vi "Read P T_NTC.vi"(7 "cjc value":dbl=25.0 format="%0.2f") -> (0 "P Set 2 Output 2":dbl format="%.3g", 1 "P Set 1 Output 2":dbl format="%.3g", 2 "mean value P":dbl, 3 "String 2":string, 6 "termopar K":dbl format="%.3g", 8 "T Set 2 Output":dbl format="%.4g", 9 "T Set 1 Output":dbl format="%.4g", 10 "mean value T":dbl, 11 "String":string)   [LabVIEW 2011]
uses:
  <vilib>/Analysis/3filter.llb/Filter Passband Type.ctl
  <vilib>/DAQmx/read.llb/DAQmx Read (Analog 1D DBL 1Chan NSamp).vi
  <vilib>/DAQmx/create/channels.llb/DAQmx Create Channel (AI-Voltage-Basic).vi
  <vilib>/DAQmx/configure/timing.llb/DAQmx Timing (Sample Clock).vi
  <vilib>/DAQmx/miscellaneous.llb/DAQmx Fill In Error Info.vi
  <vilib>/Analysis/3filter.llb/Butterworth Filter (DBL).vi
  <vilib>/Analysis/baseanly.llb/Unimode.vi
  <vilib>/Analysis/5stat.llb/RMS (DBL).vi
  <vilib>/DAQmx/create/channels.llb/DAQmx Create Channel (AI-Temperature-Thermocouple).vi
  <vilib>/Analysis/NI_AALBase.lvlib
  Program Files/National Instruments/LabVIEW 2011/resource/objmgr/daqmx.rc
  <vilib>/gmath/NI_Gmath.lvlib
  <vilib>/Analysis/NI_AALPro.lvlib
panel:
  out "output variable":dbl
  in  "input C":dbl
  in  "input B":dbl
  in  "input A":dbl
  out "Rt":dbl
  in  "Vs":dbl
  in  "intervals 3":i32=20
  in  "Statistic 3":T1(ring)
  out "P Set 1 Output 3":dbl format="%.3g"
  out "?":T2(graph)
  out "Data Set 6":dbl[](graph)
  out "?":T2(graph)
  out "Data Set 5":dbl[](graph)
  out "error 3":dbl
  in  "filter type 3":T3
  in  "high cutoff freq: fh 3":dbl=0.45000000000000007 format="%0.2f"
  in  "low cutoff freq: fl 3":dbl=0.12500000000000006 format="%0.4f"
  in  "order 3":i32=2
  out "mean value P 2":dbl
  out "String 3":string
  in  "intervals 2":i32=20
  in  "Statistic 2":T1(ring)
  out "?":T2(graph)
  out "Data Set 4":dbl[](graph)
  out "?":T2(graph)
  out "Data Set 3":dbl[](graph)
  out "error 2":dbl
  in  "filter type 2":T3
  in  "high cutoff freq: fh 2":dbl=0.45000000000000007 format="%0.2f"
  in  "low cutoff freq: fl 2":dbl=0.12500000000000006 format="%0.4f"
  in  "order 2":i32=2
  in  "intervals":i32=20
  in  "Statistic":T1(ring)
  out "?":T2(graph)
  out "Data Set 1":dbl[](graph)
  out "?":T2(graph)
  out "Data Set 2":dbl[](graph)
  out "error":dbl
  in  "filter type":T3
  in  "high cutoff freq: fh":dbl=0.45000000000000007 format="%0.2f"
  in  "low cutoff freq: fl":dbl=0.12500000000000006 format="%0.4f"
  in  "order":i32=2
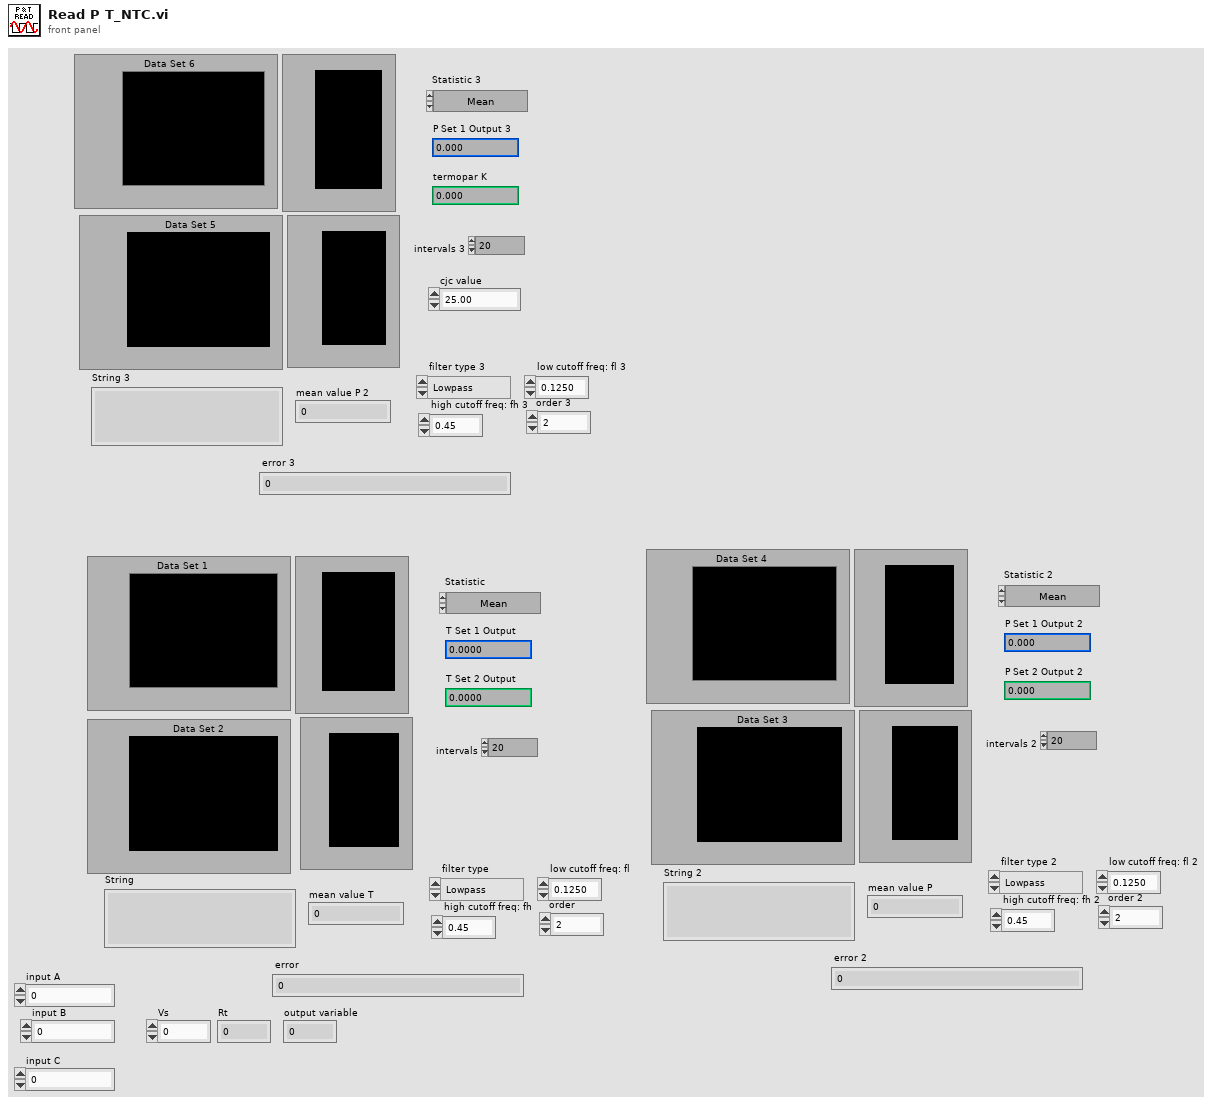
[diagram p1: front panel]
types:
  T1 = enum16{"Mean", "Standard Deviation", "Variance", "Skewness", "Kurtosis", "Median", "Mode", "RMS"}
  T2 = cluster{"Histogram: h(x)":i32[], "X Values":dbl[]}
  T3 = typedef "NI_AALBase.lvlib/Filter Passband Type.ctl" = enum32{"Lowpass", "Highpass", "Bandpass", "Bandstop"}
  T4 = enum16{"arithmetic", "geometric", "harmonic", "trimmed", "median"}
  T5 = cluster{"intervals":i32, "Statistic":enum16{"Mean", "Standard Deviation", "Variance", "Skewness", "Kurtosis", "Median", "Mode", "RMS"}}
  T6 = cluster{"intervals 2":i32, "Statistic 2":enum16{"Mean", "Standard Deviation", "Variance", "Skewness", "Kurtosis", "Median", "Mode", "RMS"}}
  T7 = cluster{"intervals 3":i32, "Statistic 3":enum16{"Mean", "Standard Deviation", "Variance", "Skewness", "Kurtosis", "Median", "Mode", "RMS"}}
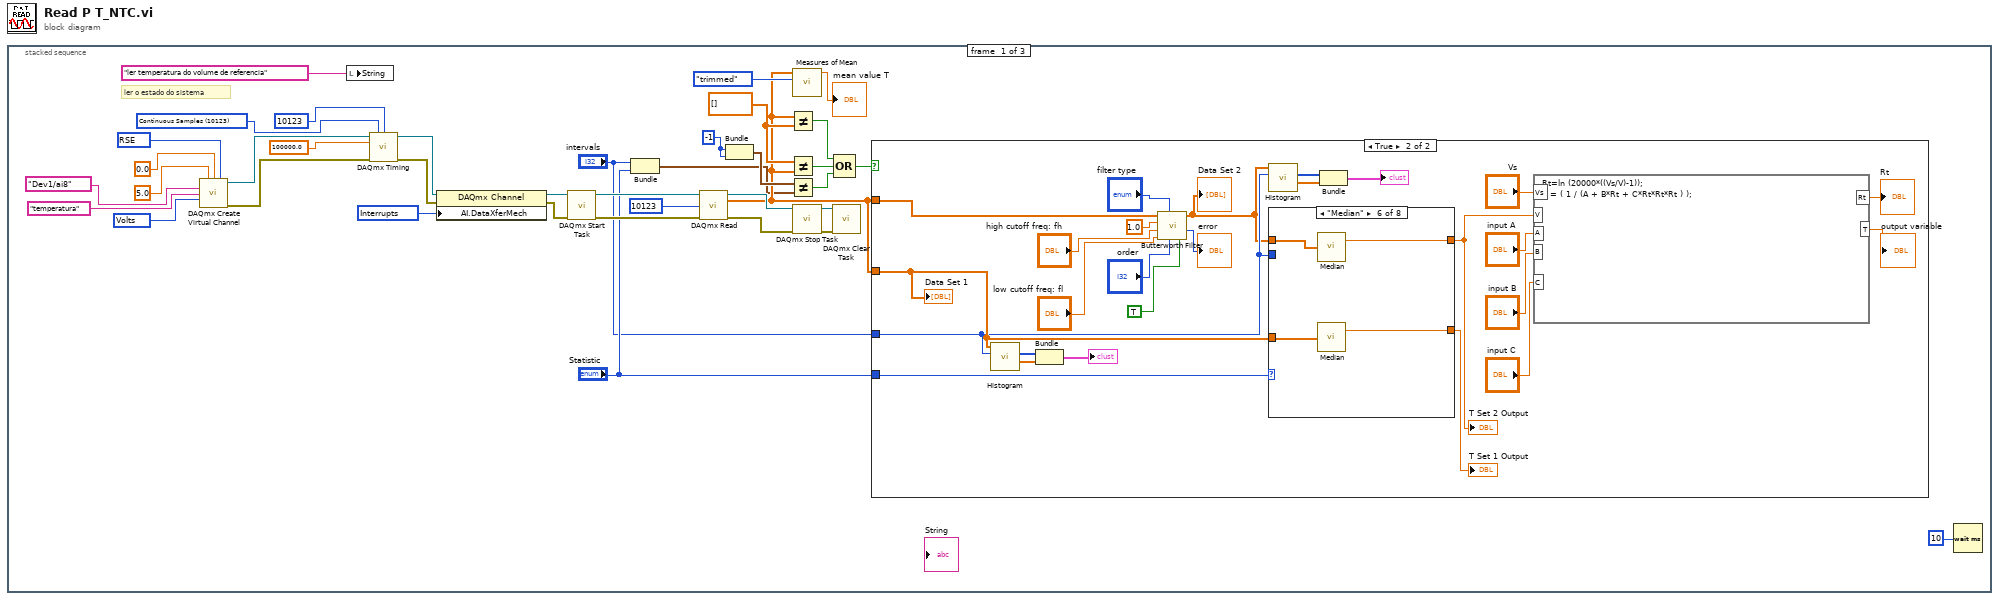
[diagram p0: block diagram]
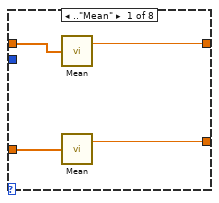
[diagram p3: hidden frame]
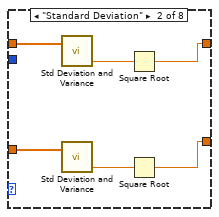
[diagram p4: hidden frame]
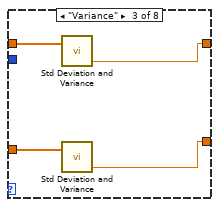
[diagram p5: hidden frame]
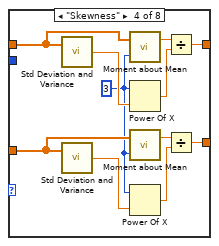
[diagram p6: hidden frame]
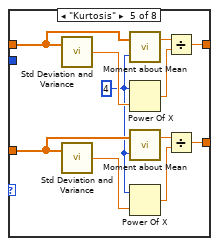
[diagram p7: hidden frame]
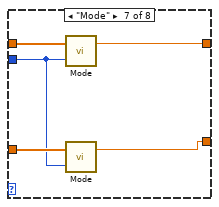
[diagram p8: hidden frame]
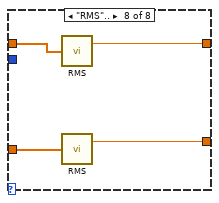
[diagram p9: hidden frame]
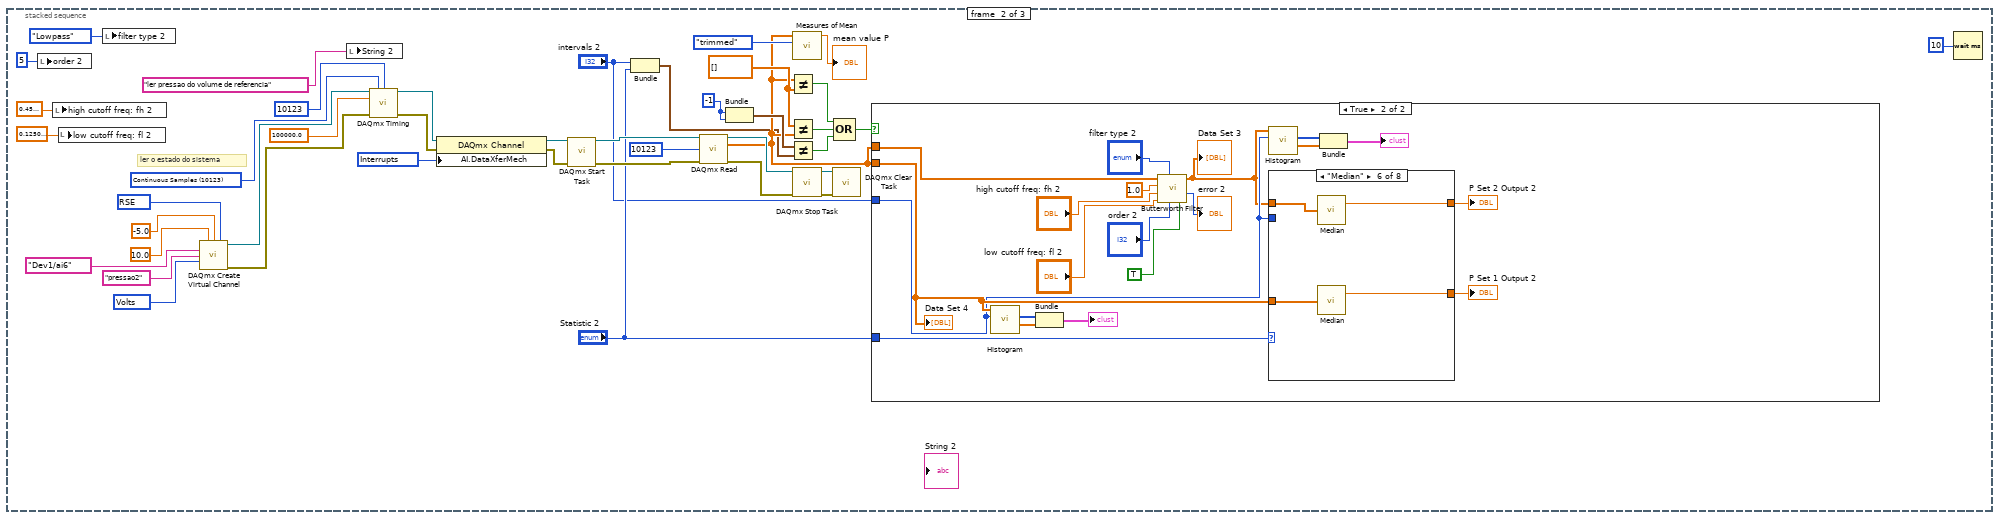
[diagram p10: hidden frame]
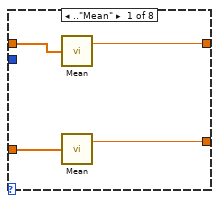
[diagram p12: hidden frame]
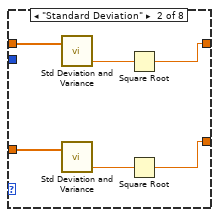
[diagram p13: hidden frame]
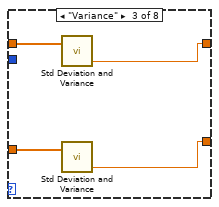
[diagram p14: hidden frame]
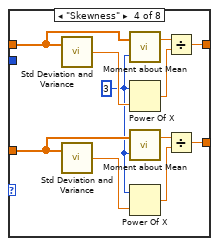
[diagram p15: hidden frame]
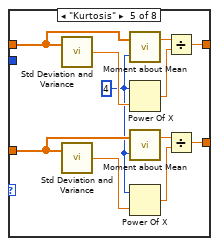
[diagram p16: hidden frame]
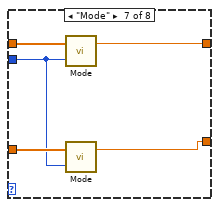
[diagram p17: hidden frame]
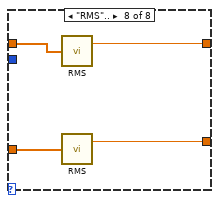
[diagram p18: hidden frame]
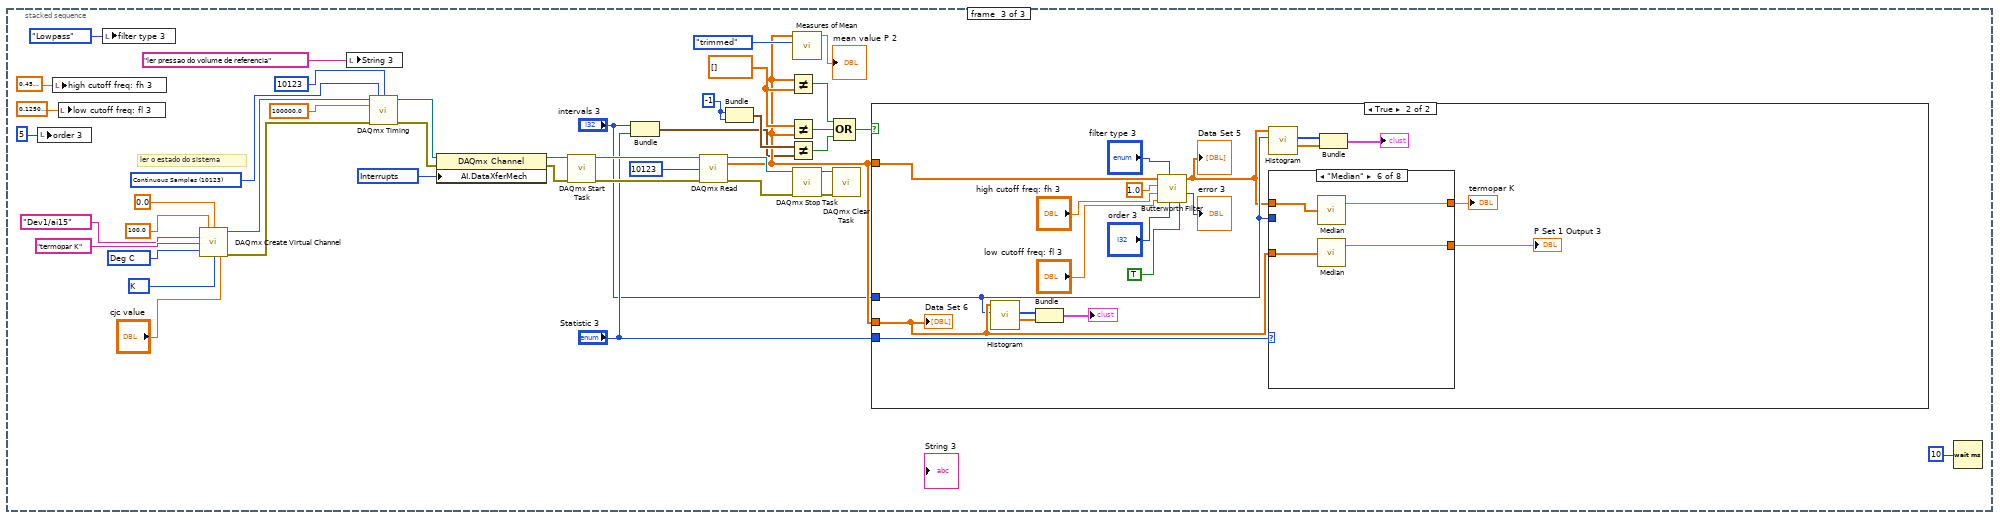
[diagram p19: hidden frame]
diagram:
  n1 = stacked-sequence {
    frame #0 {
      w34 = 10083 items=["default"=-1, "RSE"=10083, "NRSE"=10078, "Differential"=10106, "Pseudodifferential"=12529] ("input terminal configuration")
      w11 = dbl[] []
      w9 = -1
      w27 = 10204 items=["DMA"=10054, "Interrupts"=10204, "Programmed I/O"=10264, "USB Bulk"=12590] ("AI.DataXferMech")
      w30 = 10123 items=["Finite Samples"=10178, "Continuous Samples"=10123, "Hardware Timed Single Point"=12522] ("sample mode")
      w35 = 10348 items=["Volts"=10348, "From Custom Scale"=10065] ("units")
      # "ler o estado do sistema"
      n2 = call-poly <vilib>:"DAQmx Create Virtual Channel.vi"("maximum value"=5.0, "minimum value"=0.0, "input terminal configuration"=w34, "physical channels"=tag "Dev1/ai8" ("P S1"), "name to assign"="temperatura", "units"=w35) -> ("task out"=w24:refnum<k21>, "error out"=w23:errorcluster)  [unwired: 8 in]
      n3 = local write "String"("ler temperatura do volume de referencia" ("String")) -> ()
      n4 = call-poly <vilib>:"DAQmx Timing.vi"("task/channels in"=w24, "sample mode"=w30, "samples per channel"=10123, "rate"=100000.0, "error in"=w23) -> ("task out"=w29:refnum<k21>, "error out"=w28:errorcluster)  [unwired: 9 in]
      n5 = property class="DAQmx Channel"(reference=w29, error in=w28, "AI.DataXferMech"=w27) -> (reference out=w26:refnum<k21>, error out=w25:errorcluster)
      n6 = call <vilib>:"DAQmx Start Task.vi"("task/channels in"=w26, "error in"=w25) -> ("task out"=w32:refnum<k21>, "error out"=w31:errorcluster)  [unwired: 12 in]
      n7 = Bundle("intervals"="intervals", "Statistic"="Statistic") -> (w3:T5)  [unwired: 1 in]
      n8 = call-poly <vilib>:"DAQmx Read.vi"("task/channels in"=w32, "number of samples per channel"=10123, "error in"=w31) -> ("task out"=w16:refnum<k21>, "data"=w8:dbl[], "error out"=w14:errorcluster)  [unwired: 10 in]
      n9 = Bundle(w9, w9) -> (w10:cluster{i32, i32})  [unwired: 1 in]
      n10 = Not Equal?(x=w8, y=w11) -> (x != y?=w6:bool)
      n11 = Not Equal?(x=w11, y=w8) -> (x != y?=w5:bool)
      n12 = Not Equal?(x=w10, y=w3) -> (x != y?=w2:bool)
      n13 = call <vilib>:"Measures of Mean.vi"("type"=T4."trimmed", "x array"=w8) -> ("mean value"=→"mean value T":dbl)  [unwired: 8 in, 1 out]
      n14 = call <vilib>:"DAQmx Stop Task.vi"("task/channels in"=w16, "error in"=w14) -> ("task out"=w15:refnum<k21>, "error out"=w13:errorcluster)  [unwired: 12 in]
      n15 = call <vilib>:"DAQmx Clear Task.vi"("task in"=w15, "error in"=w13) -> ()  [unwired: 13 in, 1 out]
      n16 = Compound Arithmetic op=OR(w6, w5, w2) -> (w7:bool)
      n17 = case shown="True" w7 {
        tunnel: w8 -> [_ w52]
        tunnel: w8 -> [_ w61]
        tunnel: "Statistic" -> [_ w63]
        tunnel: "intervals" -> [_ w59]
        frame False {
        }
        frame True {
          n18 = call <vilib>:"Histogram.vi"("intervals"=w59, "X"=w61) -> ("X Values"=w57:dbl[], "Histogram: h(x)"=w58:i32[])  [unwired: 6 in, 2 out]
          n19 = Bundle("Histogram: h(x)"=w58, "X Values"=w57) -> (→"?":T2)  [unwired: 1 in]
          n20 = call-poly <vilib>:"Butterworth Filter.vi"("init/cont (init:F)"=TRUE, "order"="order", "filter type"="filter type", "low cutoff freq: fl"="low cutoff freq: fl", "high cutoff freq: fh"="high cutoff freq: fh", "sampling freq: fs"=1.0, "X"=w52) -> ("error"=→"error":i32, "Filtered X"=w51:dbl[])  [unwired: 1 in]
          "Data Set 2" <- w51
          n21 = call <vilib>:"Histogram.vi"("intervals"=w59, "X"=w51) -> ("X Values"=w55:dbl[], "Histogram: h(x)"=w56:i32[])  [unwired: 6 in, 2 out]
          n22 = case shown="\"Median\"" w63 {
            tunnel: w51 -> [w68 w73 w77 w84 w95 w104 w109 w113]
            tunnel: [w66 w70 w76 w81 w92 w102 w107 w112] -> w43
            tunnel: [w67 w74 w78 w85 w96 w103 w108 w111] -> w64
            tunnel: w61 -> [w65 w69 w75 w88 w99 w101 w106 w110]
            tunnel: w59 -> [_ _ _ _ _ _ w105 _]
            frame .."Mean" {
              n23 = call <vilib>:"Mean.vi"("X"=w68) -> ("mean"=w66:dbl)  [unwired: 1 out]
              n24 = call <vilib>:"Mean.vi"("X"=w65) -> ("mean"=w67:dbl)  [unwired: 1 out]
            }
            frame "Standard Deviation" {
              n25 = call <vilib>:"Std Deviation and Variance.vi"("X"=w73) -> ("variance"=w71:dbl)  [unwired: 1 in, 2 out]
              n26 = call <vilib>:"Std Deviation and Variance.vi"("X"=w69) -> ("variance"=w72:dbl)  [unwired: 1 in, 2 out]
              n27 = Square Root(x=w71) -> (sqrt(x)=w70:dbl)
              n28 = Square Root(x=w72) -> (sqrt(x)=w74:dbl)
            }
            frame "Variance" {
              n29 = call <vilib>:"Std Deviation and Variance.vi"("X"=w77) -> ("variance"=w76:dbl)  [unwired: 1 in, 2 out]
              n30 = call <vilib>:"Std Deviation and Variance.vi"("X"=w75) -> ("variance"=w78:dbl)  [unwired: 1 in, 2 out]
            }
            frame "Skewness" {
              w86 = 3
              n31 = call <vilib>:"Std Deviation and Variance.vi"("X"=w84) -> ("standard deviation"=w87:dbl)  [unwired: 1 in, 2 out]
              n32 = call <vilib>:"Std Deviation and Variance.vi"("X"=w88) -> ("standard deviation"=w89:dbl)  [unwired: 1 in, 2 out]
              n33 = call <vilib>:"Moment about Mean.vi"("order"=w86, "X"=w84) -> ("moment"=w82:dbl)  [unwired: 1 out]
              n34 = Power Of X(1:w87, 2:w86) -> (0:w83:dbl)
              n35 = call <vilib>:"Moment about Mean.vi"("order"=w86, "X"=w88) -> ("moment"=w79:dbl)  [unwired: 1 out]
              n36 = Power Of X(1:w89, 2:w86) -> (0:w80:dbl)
              n37 = Divide(x=w82, y=w83) -> (x/y=w81:dbl)
              n38 = Divide(x=w79, y=w80) -> (x/y=w85:dbl)
            }
            frame "Kurtosis" {
              w97 = 4
              n39 = call <vilib>:"Std Deviation and Variance.vi"("X"=w95) -> ("standard deviation"=w98:dbl)  [unwired: 1 in, 2 out]
              n40 = call <vilib>:"Std Deviation and Variance.vi"("X"=w99) -> ("standard deviation"=w100:dbl)  [unwired: 1 in, 2 out]
              n41 = call <vilib>:"Moment about Mean.vi"("order"=w97, "X"=w95) -> ("moment"=w93:dbl)  [unwired: 1 out]
              n42 = Power Of X(1:w98, 2:w97) -> (0:w94:dbl)
              n43 = call <vilib>:"Moment about Mean.vi"("order"=w97, "X"=w99) -> ("moment"=w91:dbl)  [unwired: 1 out]
              n44 = Power Of X(1:w100, 2:w97) -> (0:w90:dbl)
              n45 = Divide(x=w93, y=w94) -> (x/y=w92:dbl)
              n46 = Divide(x=w91, y=w90) -> (x/y=w96:dbl)
            }
            frame "Median" {
              n47 = call <vilib>:"Median.vi"("X"=w104) -> ("median"=w102:dbl)  [unwired: 1 out]
              n48 = call <vilib>:"Median.vi"("X"=w101) -> ("median"=w103:dbl)  [unwired: 1 out]
            }
            frame "Mode" {
              n49 = call-poly <vilib>:"Mode.vi"("intervals"=w105, "X"=w109) -> ("mode"=w107:dbl)  [unwired: 1 out]
              n50 = call-poly <vilib>:"Mode.vi"("intervals"=w105, "X"=w106) -> ("mode"=w108:dbl)  [unwired: 1 out]
            }
            frame "RMS".. {
              n51 = call-poly <vilib>:"RMS.vi"("X"=w113) -> ("rms value"=w112:dbl)  [unwired: 1 out]
              n52 = call-poly <vilib>:"RMS.vi"("X"=w110) -> ("rms value"=w111:dbl)  [unwired: 1 out]
            }
          }
          "T Set 1 Output" <- w64
          "T Set 2 Output" <- w43
          n53 = Bundle("Histogram: h(x)"=w56, "X Values"=w55) -> (→"?":T2)  [unwired: 1 in]
          n54 = formula code="Rt=ln (20000*((Vs/V)-1));\nT = ( 1 / (A + B*Rt + C*Rt*Rt*Rt ) );"("Vs"="Vs", "V"=w43, "A"="input A", "B"="input B", "C"="input C") -> ("Rt"=→"Rt":dbl, "T"=→"output variable":dbl)
          "Data Set 1" <- w61
        }
      }
      n55 = Wait (ms)(milliseconds to wait=u32 10) -> ()  [unwired: 1 out]
    }
    frame #1 {
      w129 = dbl[] []
      w127 = -1
      w146 = 10204 items=["DMA"=10054, "Interrupts"=10204, "Programmed I/O"=10264, "USB Bulk"=12590] ("AI.DataXferMech")
      w149 = 10123 items=["Finite Samples"=10178, "Continuous Samples"=10123, "Hardware Timed Single Point"=12522] ("sample mode")
      w153 = 10083 items=["default"=-1, "RSE"=10083, "NRSE"=10078, "Differential"=10106, "Pseudodifferential"=12529] ("input terminal configuration")
      w154 = 10348 items=["Volts"=10348, "From Custom Scale"=10065] ("units")
      # "ler o estado do sistema"
      n56 = local write "order 2"(5 ("order")) -> ()
      n57 = local write "high cutoff freq: fh 2"(0.45000000000000007 ("high cutoff freq: fh")) -> ()
      n58 = local write "low cutoff freq: fl 2"(0.12500000000000006 ("low cutoff freq: fl")) -> ()
      n59 = local write "filter type 2"(Filter_Passband_Type."Lowpass" ("filter type")) -> ()
      n60 = call-poly <vilib>:"DAQmx Create Virtual Channel.vi"("maximum value"=10.0, "minimum value"=-5.0, "input terminal configuration"=w153, "physical channels"=tag "Dev1/ai6" ("P S1"), "name to assign"="pressao2", "units"=w154) -> ("task out"=w143:refnum<k21>, "error out"=w142:errorcluster)  [unwired: 8 in]
      n61 = local write "String 2"("ler pressao do volume de referencia" ("String")) -> ()
      n62 = call-poly <vilib>:"DAQmx Timing.vi"("task/channels in"=w143, "sample mode"=w149, "samples per channel"=10123, "rate"=100000.0, "error in"=w142) -> ("task out"=w148:refnum<k21>, "error out"=w147:errorcluster)  [unwired: 9 in]
      n63 = property class="DAQmx Channel"(reference=w148, error in=w147, "AI.DataXferMech"=w146) -> (reference out=w145:refnum<k21>, error out=w144:errorcluster)
      n64 = call <vilib>:"DAQmx Start Task.vi"("task/channels in"=w145, "error in"=w144) -> ("task out"=w151:refnum<k21>, "error out"=w150:errorcluster)  [unwired: 12 in]
      n65 = Bundle("intervals 2"="intervals 2", "Statistic 2"="Statistic 2") -> (w121:T6)  [unwired: 1 in]
      n66 = call-poly <vilib>:"DAQmx Read.vi"("task/channels in"=w151, "number of samples per channel"=10123, "error in"=w150) -> ("task out"=w135:refnum<k21>, "data"=w126:dbl[], "error out"=w133:errorcluster)  [unwired: 10 in]
      n67 = Bundle(w127, w127) -> (w128:cluster{i32, i32})  [unwired: 1 in]
      n68 = Not Equal?(x=w126, y=w129) -> (x != y?=w124:bool)
      n69 = Not Equal?(x=w129, y=w126) -> (x != y?=w123:bool)
      n70 = Not Equal?(x=w128, y=w121) -> (x != y?=w120:bool)
      n71 = call <vilib>:"Measures of Mean.vi"("type"=T4."trimmed", "x array"=w126) -> ("mean value"=→"mean value P":dbl)  [unwired: 8 in, 1 out]
      n72 = call <vilib>:"DAQmx Stop Task.vi"("task/channels in"=w135, "error in"=w133) -> ("task out"=w134:refnum<k21>, "error out"=w132:errorcluster)  [unwired: 12 in]
      n73 = call <vilib>:"DAQmx Clear Task.vi"("task in"=w134, "error in"=w132) -> ()  [unwired: 13 in, 1 out]
      n74 = Compound Arithmetic op=OR(w124, w123, w120) -> (w125:bool)
      n75 = case shown="True" w125 {
        tunnel: w126 -> [_ w162]
        tunnel: w126 -> [_ w171]
        tunnel: "Statistic 2" -> [_ w173]
        tunnel: "intervals 2" -> [_ w169]
        frame False {
        }
        frame True {
          n76 = call <vilib>:"Histogram.vi"("intervals"=w169, "X"=w171) -> ("X Values"=w167:dbl[], "Histogram: h(x)"=w168:i32[])  [unwired: 6 in, 2 out]
          n77 = Bundle("Histogram: h(x)"=w168, "X Values"=w167) -> (→"?":T2)  [unwired: 1 in]
          n78 = call-poly <vilib>:"Butterworth Filter.vi"("init/cont (init:F)"=TRUE, "order"="order 2", "filter type"="filter type 2", "low cutoff freq: fl"="low cutoff freq: fl 2", "high cutoff freq: fh"="high cutoff freq: fh 2", "sampling freq: fs"=1.0, "X"=w162) -> ("error"=→"error 2":i32, "Filtered X"=w161:dbl[])  [unwired: 1 in]
          "Data Set 3" <- w161
          n79 = call <vilib>:"Histogram.vi"("intervals"=w169, "X"=w161) -> ("X Values"=w165:dbl[], "Histogram: h(x)"=w166:i32[])  [unwired: 6 in, 2 out]
          n80 = case shown="\"Median\"" w173 {
            tunnel: w161 -> [w179 w184 w188 w195 w206 w215 w220 w224]
            tunnel: [w177 w181 w187 w192 w203 w213 w218 w223] -> w174
            tunnel: [w178 w185 w189 w196 w207 w214 w219 w222] -> w175
            tunnel: w171 -> [w176 w180 w186 w199 w210 w212 w217 w221]
            tunnel: w169 -> [_ _ _ _ _ _ w216 _]
            frame .."Mean" {
              n81 = call <vilib>:"Mean.vi"("X"=w179) -> ("mean"=w177:dbl)  [unwired: 1 out]
              n82 = call <vilib>:"Mean.vi"("X"=w176) -> ("mean"=w178:dbl)  [unwired: 1 out]
            }
            frame "Standard Deviation" {
              n83 = call <vilib>:"Std Deviation and Variance.vi"("X"=w184) -> ("variance"=w182:dbl)  [unwired: 1 in, 2 out]
              n84 = call <vilib>:"Std Deviation and Variance.vi"("X"=w180) -> ("variance"=w183:dbl)  [unwired: 1 in, 2 out]
              n85 = Square Root(x=w182) -> (sqrt(x)=w181:dbl)
              n86 = Square Root(x=w183) -> (sqrt(x)=w185:dbl)
            }
            frame "Variance" {
              n87 = call <vilib>:"Std Deviation and Variance.vi"("X"=w188) -> ("variance"=w187:dbl)  [unwired: 1 in, 2 out]
              n88 = call <vilib>:"Std Deviation and Variance.vi"("X"=w186) -> ("variance"=w189:dbl)  [unwired: 1 in, 2 out]
            }
            frame "Skewness" {
              w197 = 3
              n89 = call <vilib>:"Std Deviation and Variance.vi"("X"=w195) -> ("standard deviation"=w198:dbl)  [unwired: 1 in, 2 out]
              n90 = call <vilib>:"Std Deviation and Variance.vi"("X"=w199) -> ("standard deviation"=w200:dbl)  [unwired: 1 in, 2 out]
              n91 = call <vilib>:"Moment about Mean.vi"("order"=w197, "X"=w195) -> ("moment"=w193:dbl)  [unwired: 1 out]
              n92 = Power Of X(1:w198, 2:w197) -> (0:w194:dbl)
              n93 = call <vilib>:"Moment about Mean.vi"("order"=w197, "X"=w199) -> ("moment"=w190:dbl)  [unwired: 1 out]
              n94 = Power Of X(1:w200, 2:w197) -> (0:w191:dbl)
              n95 = Divide(x=w193, y=w194) -> (x/y=w192:dbl)
              n96 = Divide(x=w190, y=w191) -> (x/y=w196:dbl)
            }
            frame "Kurtosis" {
              w208 = 4
              n97 = call <vilib>:"Std Deviation and Variance.vi"("X"=w206) -> ("standard deviation"=w209:dbl)  [unwired: 1 in, 2 out]
              n98 = call <vilib>:"Std Deviation and Variance.vi"("X"=w210) -> ("standard deviation"=w211:dbl)  [unwired: 1 in, 2 out]
              n99 = call <vilib>:"Moment about Mean.vi"("order"=w208, "X"=w206) -> ("moment"=w204:dbl)  [unwired: 1 out]
              n100 = Power Of X(1:w209, 2:w208) -> (0:w205:dbl)
              n101 = call <vilib>:"Moment about Mean.vi"("order"=w208, "X"=w210) -> ("moment"=w202:dbl)  [unwired: 1 out]
              n102 = Power Of X(1:w211, 2:w208) -> (0:w201:dbl)
              n103 = Divide(x=w204, y=w205) -> (x/y=w203:dbl)
              n104 = Divide(x=w202, y=w201) -> (x/y=w207:dbl)
            }
            frame "Median" {
              n105 = call <vilib>:"Median.vi"("X"=w215) -> ("median"=w213:dbl)  [unwired: 1 out]
              n106 = call <vilib>:"Median.vi"("X"=w212) -> ("median"=w214:dbl)  [unwired: 1 out]
            }
            frame "Mode" {
              n107 = call-poly <vilib>:"Mode.vi"("intervals"=w216, "X"=w220) -> ("mode"=w218:dbl)  [unwired: 1 out]
              n108 = call-poly <vilib>:"Mode.vi"("intervals"=w216, "X"=w217) -> ("mode"=w219:dbl)  [unwired: 1 out]
            }
            frame "RMS".. {
              n109 = call-poly <vilib>:"RMS.vi"("X"=w224) -> ("rms value"=w223:dbl)  [unwired: 1 out]
              n110 = call-poly <vilib>:"RMS.vi"("X"=w221) -> ("rms value"=w222:dbl)  [unwired: 1 out]
            }
          }
          "P Set 1 Output 2" <- w175
          "P Set 2 Output 2" <- w174
          n111 = Bundle("Histogram: h(x)"=w166, "X Values"=w165) -> (→"?":T2)  [unwired: 1 in]
          "Data Set 4" <- w171
        }
      }
      n112 = Wait (ms)(milliseconds to wait=u32 10) -> ()  [unwired: 1 out]
    }
    frame #2 {
      w228 = 10073 items=["J"=10072, "K"=10073, "N"=10077, "R"=10082, "S"=10085, "T"=10086, "B"=10047, "E"=10055] ("thermocouple type")
      w229 = 10143 items=["Deg C"=10143, "Deg F"=10144, "Kelvins"=10325, "Deg R"=10145, "From Custom Scale"=10065] ("units")
      w245 = dbl[] []
      w243 = -1
      w260 = 10204 items=["DMA"=10054, "Interrupts"=10204, "Programmed I/O"=10264, "USB Bulk"=12590] ("AI.DataXferMech")
      w263 = 10123 items=["Finite Samples"=10178, "Continuous Samples"=10123, "Hardware Timed Single Point"=12522] ("sample mode")
      # "ler o estado do sistema"
      n113 = local write "order 3"(5 ("order")) -> ()
      n114 = local write "high cutoff freq: fh 3"(0.45000000000000007 ("high cutoff freq: fh")) -> ()
      n115 = local write "low cutoff freq: fl 3"(0.12500000000000006 ("low cutoff freq: fl")) -> ()
      n116 = local write "filter type 3"(Filter_Passband_Type."Lowpass" ("filter type")) -> ()
      n117 = call-poly <vilib>:"DAQmx Create Virtual Channel.vi"("maximum value"=100.0, "minimum value"=0.0, "physical channels"=tag "Dev1/ai15" ("P S1"), "name to assign"="termopar K", "units"=w229, "thermocouple type"=w228, "cjc value"="cjc value") -> ("task out"=w257:refnum<k21>, "error out"=w256:errorcluster)  [unwired: 7 in]
      n118 = local write "String 3"("ler pressao do volume de referencia" ("String")) -> ()
      n119 = call-poly <vilib>:"DAQmx Timing.vi"("task/channels in"=w257, "sample mode"=w263, "samples per channel"=10123, "rate"=100000.0, "error in"=w256) -> ("task out"=w262:refnum<k21>, "error out"=w261:errorcluster)  [unwired: 9 in]
      n120 = property class="DAQmx Channel"(reference=w262, error in=w261, "AI.DataXferMech"=w260) -> (reference out=w259:refnum<k21>, error out=w258:errorcluster)
      n121 = call <vilib>:"DAQmx Start Task.vi"("task/channels in"=w259, "error in"=w258) -> ("task out"=w265:refnum<k21>, "error out"=w264:errorcluster)  [unwired: 12 in]
      n122 = Bundle("intervals 3"="intervals 3", "Statistic 3"="Statistic 3") -> (w237:T7)  [unwired: 1 in]
      n123 = call-poly <vilib>:"DAQmx Read.vi"("task/channels in"=w265, "number of samples per channel"=10123, "error in"=w264) -> ("task out"=w251:refnum<k21>, "data"=w242:dbl[], "error out"=w249:errorcluster)  [unwired: 10 in]
      n124 = Bundle(w243, w243) -> (w244:cluster{i32, i32})  [unwired: 1 in]
      n125 = Not Equal?(x=w242, y=w245) -> (x != y?=w240:bool)
      n126 = Not Equal?(x=w245, y=w242) -> (x != y?=w239:bool)
      n127 = Not Equal?(x=w244, y=w237) -> (x != y?=w236:bool)
      n128 = call <vilib>:"Measures of Mean.vi"("type"=T4."trimmed", "x array"=w242) -> ("mean value"=→"mean value P 2":dbl)  [unwired: 8 in, 1 out]
      n129 = call <vilib>:"DAQmx Stop Task.vi"("task/channels in"=w251, "error in"=w249) -> ("task out"=w250:refnum<k21>, "error out"=w248:errorcluster)  [unwired: 12 in]
      n130 = call <vilib>:"DAQmx Clear Task.vi"("task in"=w250, "error in"=w248) -> ()  [unwired: 13 in, 1 out]
      n131 = Compound Arithmetic op=OR(w240, w239, w236) -> (w241:bool)
      n132 = case shown="True" w241 {
        tunnel: w242 -> [_ w274]
        tunnel: w242 -> [_ w283]
        tunnel: "Statistic 3" -> [_ w285]
        tunnel: "intervals 3" -> [_ w281]
        frame False {
        }
        frame True {
          n133 = call <vilib>:"Histogram.vi"("intervals"=w281, "X"=w283) -> ("X Values"=w279:dbl[], "Histogram: h(x)"=w280:i32[])  [unwired: 6 in, 2 out]
          n134 = Bundle("Histogram: h(x)"=w280, "X Values"=w279) -> (→"?":T2)  [unwired: 1 in]
          n135 = call-poly <vilib>:"Butterworth Filter.vi"("init/cont (init:F)"=TRUE, "order"="order 3", "filter type"="filter type 3", "low cutoff freq: fl"="low cutoff freq: fl 3", "high cutoff freq: fh"="high cutoff freq: fh 3", "sampling freq: fs"=1.0, "X"=w274) -> ("error"=→"error 3":i32, "Filtered X"=w273:dbl[])  [unwired: 1 in]
          "Data Set 5" <- w273
          n136 = call <vilib>:"Histogram.vi"("intervals"=w281, "X"=w273) -> ("X Values"=w277:dbl[], "Histogram: h(x)"=w278:i32[])  [unwired: 6 in, 2 out]
          n137 = case shown="\"Median\"" w285 {
            tunnel: w273 -> [w291 w296 w300 w307 w318 w327 w332 w336]
            tunnel: [w289 w293 w299 w304 w315 w325 w330 w335] -> w286
            tunnel: [w290 w297 w301 w308 w319 w326 w331 w334] -> w287
            tunnel: w283 -> [w288 w292 w298 w311 w322 w324 w329 w333]
            tunnel: w281 -> [_ _ _ _ _ _ w328 _]
            frame .."Mean" {
              n138 = call <vilib>:"Mean.vi"("X"=w291) -> ("mean"=w289:dbl)  [unwired: 1 out]
              n139 = call <vilib>:"Mean.vi"("X"=w288) -> ("mean"=w290:dbl)  [unwired: 1 out]
            }
            frame "Standard Deviation" {
              n140 = call <vilib>:"Std Deviation and Variance.vi"("X"=w296) -> ("variance"=w294:dbl)  [unwired: 1 in, 2 out]
              n141 = call <vilib>:"Std Deviation and Variance.vi"("X"=w292) -> ("variance"=w295:dbl)  [unwired: 1 in, 2 out]
              n142 = Square Root(x=w294) -> (sqrt(x)=w293:dbl)
              n143 = Square Root(x=w295) -> (sqrt(x)=w297:dbl)
            }
            frame "Variance" {
              n144 = call <vilib>:"Std Deviation and Variance.vi"("X"=w300) -> ("variance"=w299:dbl)  [unwired: 1 in, 2 out]
              n145 = call <vilib>:"Std Deviation and Variance.vi"("X"=w298) -> ("variance"=w301:dbl)  [unwired: 1 in, 2 out]
            }
            frame "Skewness" {
              w309 = 3
              n146 = call <vilib>:"Std Deviation and Variance.vi"("X"=w307) -> ("standard deviation"=w310:dbl)  [unwired: 1 in, 2 out]
              n147 = call <vilib>:"Std Deviation and Variance.vi"("X"=w311) -> ("standard deviation"=w312:dbl)  [unwired: 1 in, 2 out]
              n148 = call <vilib>:"Moment about Mean.vi"("order"=w309, "X"=w307) -> ("moment"=w305:dbl)  [unwired: 1 out]
              n149 = Power Of X(1:w310, 2:w309) -> (0:w306:dbl)
              n150 = call <vilib>:"Moment about Mean.vi"("order"=w309, "X"=w311) -> ("moment"=w302:dbl)  [unwired: 1 out]
              n151 = Power Of X(1:w312, 2:w309) -> (0:w303:dbl)
              n152 = Divide(x=w305, y=w306) -> (x/y=w304:dbl)
              n153 = Divide(x=w302, y=w303) -> (x/y=w308:dbl)
            }
            frame "Kurtosis" {
              w320 = 4
              n154 = call <vilib>:"Std Deviation and Variance.vi"("X"=w318) -> ("standard deviation"=w321:dbl)  [unwired: 1 in, 2 out]
              n155 = call <vilib>:"Std Deviation and Variance.vi"("X"=w322) -> ("standard deviation"=w323:dbl)  [unwired: 1 in, 2 out]
              n156 = call <vilib>:"Moment about Mean.vi"("order"=w320, "X"=w318) -> ("moment"=w316:dbl)  [unwired: 1 out]
              n157 = Power Of X(1:w321, 2:w320) -> (0:w317:dbl)
              n158 = call <vilib>:"Moment about Mean.vi"("order"=w320, "X"=w322) -> ("moment"=w314:dbl)  [unwired: 1 out]
              n159 = Power Of X(1:w323, 2:w320) -> (0:w313:dbl)
              n160 = Divide(x=w316, y=w317) -> (x/y=w315:dbl)
              n161 = Divide(x=w314, y=w313) -> (x/y=w319:dbl)
            }
            frame "Median" {
              n162 = call <vilib>:"Median.vi"("X"=w327) -> ("median"=w325:dbl)  [unwired: 1 out]
              n163 = call <vilib>:"Median.vi"("X"=w324) -> ("median"=w326:dbl)  [unwired: 1 out]
            }
            frame "Mode" {
              n164 = call-poly <vilib>:"Mode.vi"("intervals"=w328, "X"=w332) -> ("mode"=w330:dbl)  [unwired: 1 out]
              n165 = call-poly <vilib>:"Mode.vi"("intervals"=w328, "X"=w329) -> ("mode"=w331:dbl)  [unwired: 1 out]
            }
            frame "RMS".. {
              n166 = call-poly <vilib>:"RMS.vi"("X"=w336) -> ("rms value"=w335:dbl)  [unwired: 1 out]
              n167 = call-poly <vilib>:"RMS.vi"("X"=w333) -> ("rms value"=w334:dbl)  [unwired: 1 out]
            }
          }
          "P Set 1 Output 3" <- w287
          "termopar K" <- w286
          n168 = Bundle("Histogram: h(x)"=w278, "X Values"=w277) -> (→"?":T2)  [unwired: 1 in]
          "Data Set 6" <- w283
        }
      }
      n169 = Wait (ms)(milliseconds to wait=u32 10) -> ()  [unwired: 1 out]
    }
  }
